vi "Find And Replace All VIs.vi"(6 "Total Iteration Progress":dbl, 7 "Project":refnum<vi>, 8 "error in (no error)":errorcluster, 10 "MetaDataObj":refnum<class "MetaDataObj.lvclass">, 11 "VI References":refnum<vi>[](array[refnum])) -> (0 "error out":errorcluster, 3 "dup VI References":refnum<vi>[](array[refnum]))   [LabVIEW 2016, in "MetaDataObj.lvclass"]
uses:
  <resource>/dialog/NewProjectWizard/MetaDataObj/MetaDataObj.lvclass
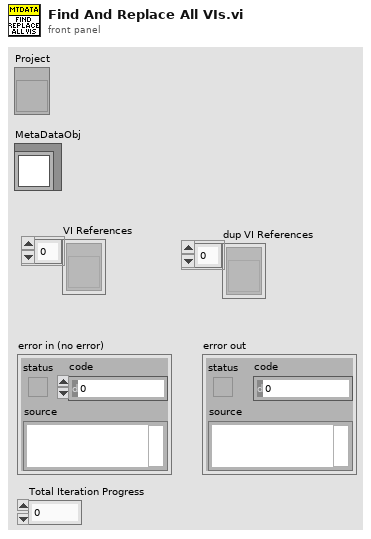
[diagram p1: front panel]
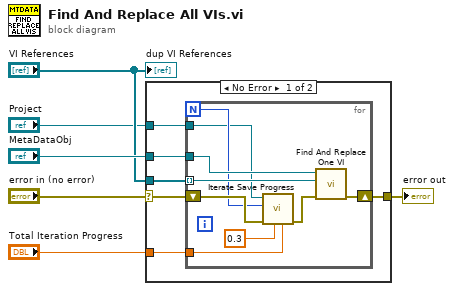
[diagram p0: block diagram]
diagram:
  n1 = case shown="No Error" "error in (no error)" {
    selector: "error in (no error)" -> [w9 w22]
    tunnel: "MetaDataObj" -> [w12 _]
    tunnel: [w11 w22] -> w5
    tunnel: "VI References" -> [w10 _]
    tunnel: "Total Iteration Progress" -> [w8 _]
    tunnel: "Project" -> [w7 _]
    frame No Error {
      n2 = for {
        N -> [w15]
        tunnel: w10 -> [w21] mode=indexing
        shift-right: [w20] -> w11
        shift-left: w9 -> [w18]
        tunnel: w12 -> [w19]
        tunnel: w8 -> [w14]
        tunnel: w7 -> [w13]
        n3 = call <resource>:"Iterate Save Progress.vi"("Total Iteration Progress"=w14, "This Task's Percentage"=0.3, "error in (no error)"=w18, "Total Iterations (this task)"=w15, "Project"=w13) -> ("error out"=w17:errorcluster)  [unwired: 6 in]
        n4 = call <resource>:"Find And Replace One VI.vi"("error in (no error)"=w17, "VI Ref in"=w21, "MetaDataObj"=w19) -> ("error out"=w20:errorcluster)  [unwired: 7 in, 1 out]
      }
    }
    frame Error {
    }
  }
  "error out" <- w5
  "dup VI References" <- "VI References"
